vi "N channel Pulse and Transition Measurements.vi"() -> ()   [LabVIEW 2023]
doc: "This example demonstrates how to use the N Channel pulse and transition measurement VIs to measure the data from a maximum of three channels."
uses:
  <vilib>/measure/mascope.llb/Transition Measurements N chan.vi
  <vilib>/measure/mascope.llb/Pulse Measurements N chan.vi
  <vilib>/measure/mascope.llb/Cycle Average and RMS N chan.vi
  <vilib>/measure/mascope.llb/Amplitude and Levels N chan.vi
  <vilib>/measure/NI_MAPro.lvlib
  <vilib>/measure/NI_MABase.lvlib
panel:
  out "Simulated Data":waveform(dbl)[](graph)
  in  "Measurements":T1(tab)
  out "undershoots":dbl[](array[numeric])
  out "overshoots":dbl[](array[numeric])
  out "duty cycle":dbl[](array[numeric])
  out "pulse duration":dbl[](array[numeric])
  out "period":dbl[](array[numeric])
  out "cycle RMS":dbl[](array[numeric])
  out "cycle average":dbl[](array[numeric])
  out "low state level":dbl[](array[numeric])
  out "high state level":dbl[](array[numeric])
  out "amplitude":dbl[](array[numeric])
  in  "Stop":bool
  # "Overview: Demonstrates how to use several different Waveform Measurements VIs to perform measurements on multiple channels.\nRequirements: LabVIEW Full Development System\nInstructions:\n1. Run the VI.\n2. Select different tabs on the tab control to perform different measurements on the Simulated Data.\n3. Click Stop to stop the VI."
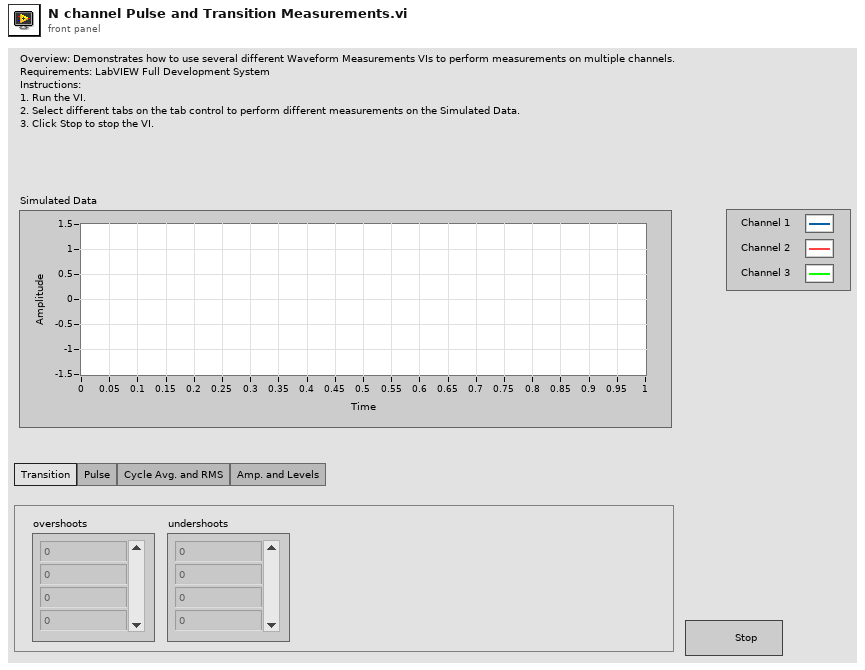
[diagram p1: front panel]
types:
  T1 = enum32{"Transition", "Pulse", "Cycle Avg. and RMS", "Amp. and Levels"}
  T2 = enum16{"Sine Wave", "Triangle Wave", "Square Wave", "Sawtooth Wave"}
  T3 = cluster{"undershoot (%)":dbl, "overshoot (%)":dbl}[]
  T4 = cluster{"undershoot (%)":dbl, "overshoot (%)":dbl}
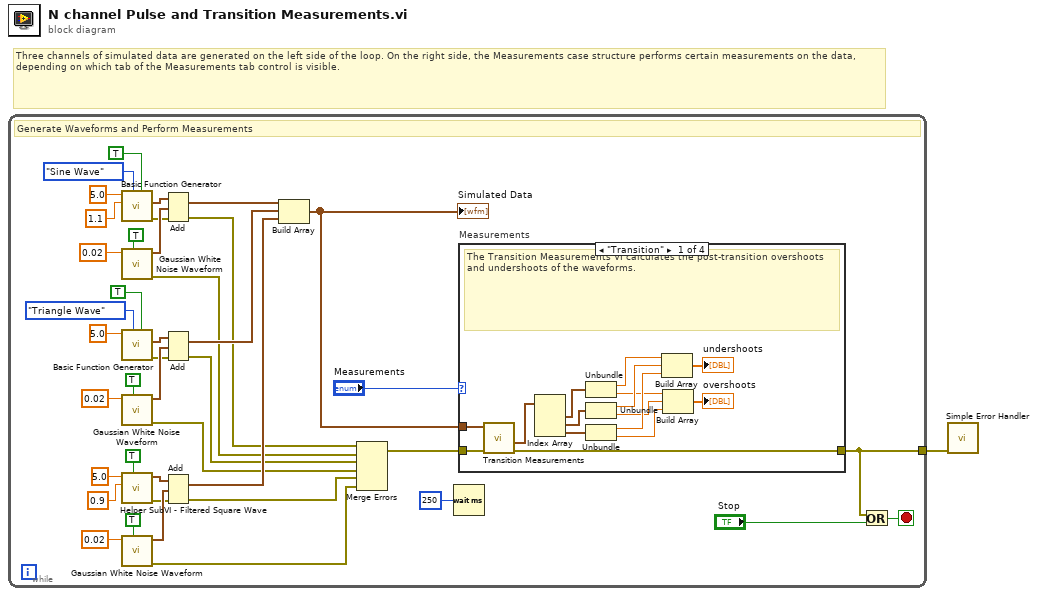
[diagram p0: block diagram]
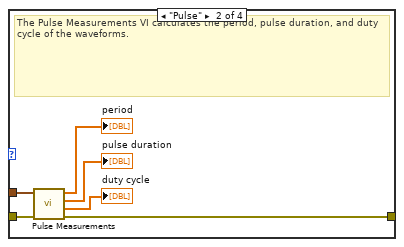
[diagram p2: hidden frame]
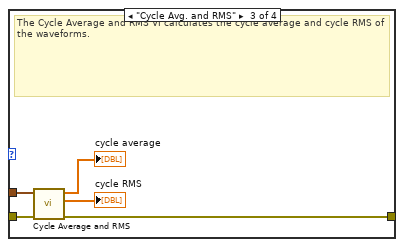
[diagram p3: hidden frame]
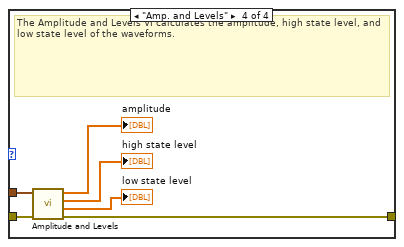
[diagram p4: hidden frame]
diagram:
  # "Three channels of simulated data are generated on the left side of the loop. On the right side, the Measurements case structure performs certain measurements on the data, depending on which tab of the Measurements tab control is visible."
  n1 = while {
    tunnel: [w38] -> w1
    stop <- w40 stop-if-true
    # "Generate Waveforms and Perform Measurements"
    n2 = call <vilib>:"Basic Function Generator.vi"("reset signal"=TRUE, "signal type"=T2."Sine Wave", "amplitude"=1.1, "frequency"=5.0) -> ("error out"=w13:errorcluster, "signal out"=w32:waveform(dbl))  [unwired: 5 in, 1 out]
    n3 = call <vilib>:"Gaussian White Noise Waveform.vi"("reset signal"=TRUE, "standard deviation"=0.02) -> ("error out"=w10:errorcluster, "signal out"=w31:waveform(dbl))  [unwired: 8 in]
    n4 = call <vilib>:"Basic Function Generator.vi"("reset signal"=TRUE, "signal type"=T2."Triangle Wave", "frequency"=5.0) -> ("error out"=w9:errorcluster, "signal out"=w26:waveform(dbl))  [unwired: 6 in, 1 out]
    n5 = call <vilib>:"Gaussian White Noise Waveform.vi"("reset signal"=TRUE, "standard deviation"=0.02) -> ("error out"=w7:errorcluster, "signal out"=w25:waveform(dbl))  [unwired: 8 in]
    n6 = call "Helper SubVI - Filtered Square Wave.vi"("reset signal"=TRUE, "signal amplitude"=0.9, "frequency"=5.0) -> ("error out"=w5:errorcluster, "Filtered Square Wave"=w21:waveform(dbl))  [unwired: 7 in]
    n7 = call <vilib>:"Gaussian White Noise Waveform.vi"("reset signal"=TRUE, "standard deviation"=0.02) -> ("error out"=w3:errorcluster, "signal out"=w22:waveform(dbl))  [unwired: 8 in]
    n8 = Add(1:w31, 2:w32, 4:w13) -> (0:w18:waveform(dbl), 3:w11:errorcluster)
    n9 = Add(1:w25, 2:w26, 4:w9) -> (0:w17:waveform(dbl), 3:w8:errorcluster)
    n10 = Add(1:w22, 2:w21, 4:w5) -> (0:w16:waveform(dbl), 3:w4:errorcluster)
    n11 = Build Array(w18, w17, w16) -> (w15:waveform(dbl)[])
    "Simulated Data" <- w15
    n12 = Merge Errors(w11, w10, w8, w7, w4, w3) -> (w14:errorcluster)
    n13 = Wait (ms)(milliseconds to wait=u32 250) -> ()  [unwired: 1 out]
    n14 = case "Measurements" shown="\"Transition\"" "Measurements" {
      tunnel: w15 -> [w57 w63 w68 w74]
      tunnel: [w56 w62 w67 w73] -> w38
      tunnel: w14 -> [w55 w61 w66 w72]
      frame "Transition" {
        # "The Transition Measurements VI calculates the post-transition overshoots and undershoots of the waveforms."
        n15 = call-poly <vilib>:"Transition Measurements.vi"("error in (no error)"=w55, "signal(s) in"=w57) -> ("error out"=w56:errorcluster, "post-transition"=w54:T3)  [unwired: 4 in, 4 out]
        n16 = Index Array(array=w54) -> (element #1=w53:T4, element #2=w52:T4, element #3=w51:T4)  [unwired: 3 in]
        n17 = Unbundle(w53) -> ("undershoot (%)"=w50:dbl, "overshoot (%)"=w47:dbl)
        n18 = Unbundle(w52) -> ("undershoot (%)"=w49:dbl, "overshoot (%)"=w46:dbl)
        n19 = Unbundle(w51) -> ("undershoot (%)"=w48:dbl, "overshoot (%)"=w45:dbl)
        n20 = Build Array(w50, w49, w48) -> (→"undershoots":dbl[])
        n21 = Build Array(w47, w46, w45) -> (→"overshoots":dbl[])
      }
      frame "Pulse" {
        # "The Pulse Measurements VI calculates the period, pulse duration, and duty cycle of the waveforms."
        n22 = call-poly <vilib>:"Pulse Measurements.vi"("error in (no error)"=w61, "signal(s) in"=w63) -> ("error out"=w62:errorcluster, "duty cycle"=→"duty cycle":dbl[], "pulse duration"=→"pulse duration":dbl[], "period"=→"period":dbl[])  [unwired: 5 in, 1 out]
      }
      frame "Cycle Avg. and RMS" {
        # "The Cycle Average and RMS VI calculates the cycle average and cycle RMS of the waveforms."
        n23 = call-poly <vilib>:"Cycle Average and RMS.vi"("error in (no error)"=w66, "signal(s) in"=w68) -> ("error out"=w67:errorcluster, "cycle RMS"=→"cycle RMS":dbl[], "cycle average"=→"cycle average":dbl[])  [unwired: 6 in, 1 out]
      }
      frame "Amp. and Levels" {
        # "The Amplitude and Levels VI calculates the amplitude, high state level, and low state level of the waveforms."
        n24 = call-poly <vilib>:"Amplitude and Levels.vi"("error in (no error)"=w72, "signal(s) in"=w74) -> ("error out"=w73:errorcluster, "low state level"=→"low state level":dbl[], "high state level"=→"high state level":dbl[], "amplitude"=→"amplitude":dbl[])  [unwired: 6 in]
      }
    }
    n25 = Or(x=w38, y="Stop") -> (x .or. y?=w40:bool)
  }
  n26 = call <vilib>:"Simple Error Handler.vi"("error in (no error)"=w1) -> ()  [unwired: 4 in, 5 out]
